vi "Nav Joystick read module.vi"(3 "error in":errorcluster) -> (7 "Forward":dbl(slide) scale=-10.0..10.0, 8 "Heading":dbl(slide) scale=-10.0..10.0, 9 "Lat":dbl(slide) scale=-10.0..10.0, 10 "error out":errorcluster)   [LabVIEW 2021]
doc: "Demonstrates how to access assembly instance data by using Explicit Messaging."
panel:
  out "Trim":u8(slide) scale=0.0..255.0
  out "Right":bool
  out "Left":bool
  out "depth":bool
  out "Dn":bool
  out "Up":bool
  out "element":u8
  out "data received":u8[](array[numeric])
  in  "network path":string="192.168.81.28"
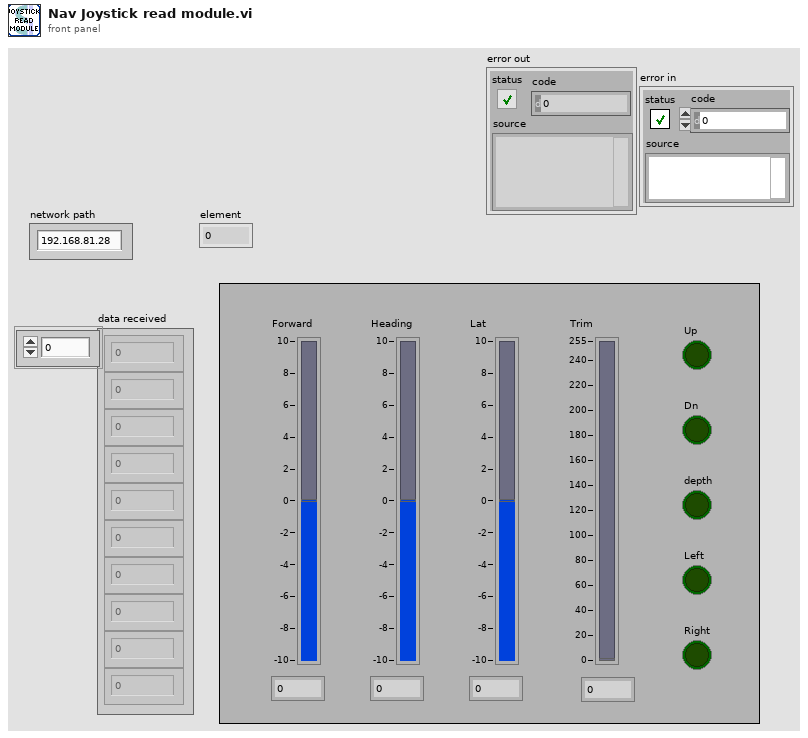
[diagram p1: front panel]
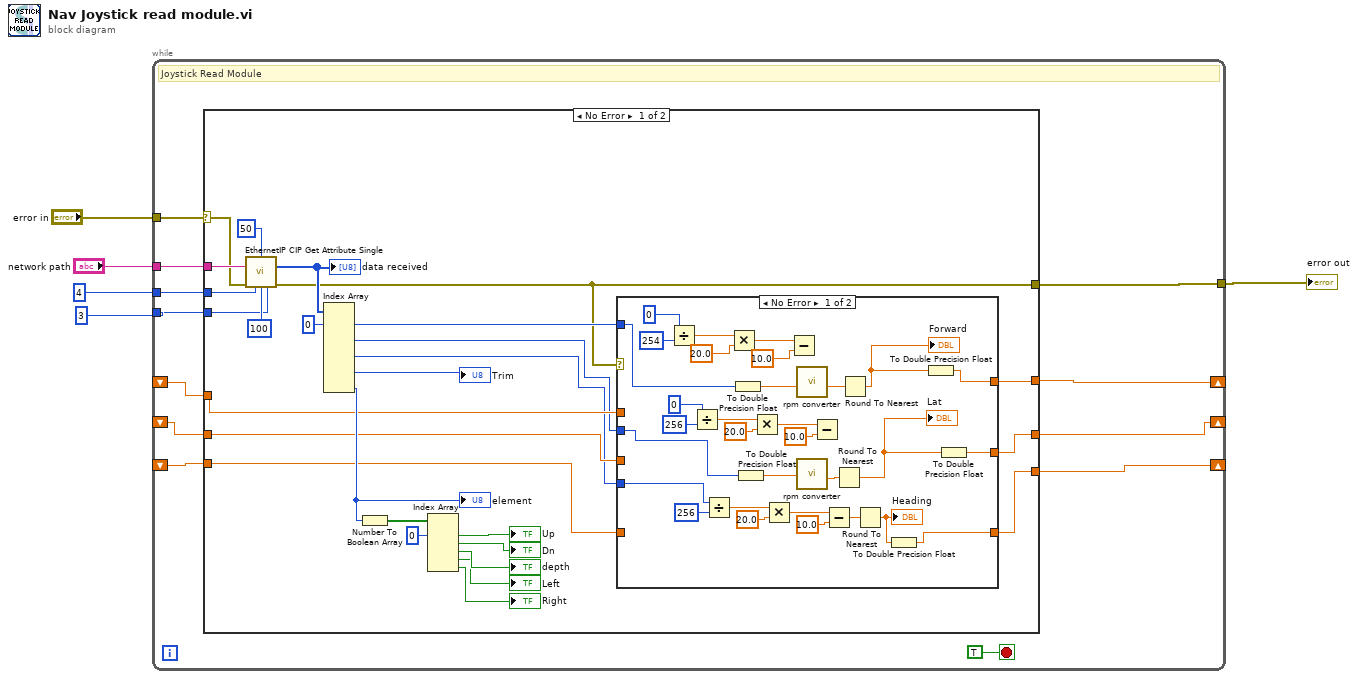
[diagram p0: block diagram]
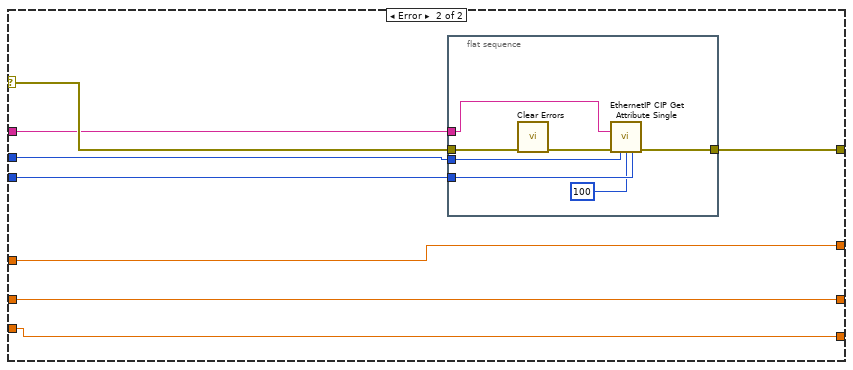
[diagram p3: hidden frame]
diagram:
  n1 = while {
    tunnel: "network path" -> [w17]
    tunnel: 4 ("Class") -> [w16]
    tunnel: 3 ("Attribute") -> [w15]
    shift-right: [w10] -> _
    shift-left: _ -> [w11]
    tunnel: "error in" -> [w12]
    tunnel: [w14] -> w2
    shift-right: [w9] -> _
    shift-left: _ -> [w8]
    shift-right: [w6] -> _
    shift-left: _ -> [w7]
    stop <- TRUE stop-if-true
    # "Joystick Read Module"
    n2 = case shown="No Error" w12 {
      selector: w12 -> [w18 w86]
      tunnel: w17 -> [w43 w84]
      tunnel: w16 -> [w42 w83]
      tunnel: w15 -> [w41 w82]
      tunnel: [w26 w85] -> w14
      tunnel: [w27 w81] -> w10
      tunnel: w11 -> [w25 w81]
      tunnel: [w24 w80] -> w9
      tunnel: w8 -> [w23 w80]
      tunnel: w7 -> [w21 w79]
      tunnel: [w20 w79] -> w6
      frame No Error {
        n3 = call <vilib>:"EthernetIP CIP Get Attribute Single.vi"("Timeout (ms)"=50 ("timeout [ms]"), "Network Path"=w43, "error in"=w18, "Class"=w42, "Instance"=u32 100 ("assembly instance ID"), "Attribute"=w41) -> ("Data"=w39:u8[], "error out"=w26:errorcluster)  [unwired: 1 in, 7 out]
        "data received" <- w39
        n4 = Index Array(array=w39, index #1=0 ("index")) -> (element #1=w28:u8, element #3=w22:u8, element #5=w19:u8, element #7=→"Trim":u8, element #9=w37:u8)  [unwired: 8 in, 4 out]
        "element" <- w37
        n5 = Number To Boolean Array(number=w37) -> (Boolean array=w36:bool[])
        n6 = Index Array(array=w36, index #1=0 ("index")) -> (element #1=→"Up":bool, element #2=→"Dn":bool, element #3=→"depth":bool, element #4=→"Left":bool, element #5=→"Right":bool)  [unwired: 4 in]
        n7 = case shown="No Error" w26 {
          tunnel: w28 -> [w51 _]
          tunnel: [w69 w78] -> w27
          tunnel: w25 -> [_ w78]
          tunnel: [w62 w77] -> w24
          tunnel: w23 -> [_ w77]
          tunnel: w22 -> [w48 _]
          tunnel: [w54 w76] -> w20
          tunnel: w21 -> [_ w76]
          tunnel: w19 -> [w53 _]
          frame No Error {
            n8 = Divide(x=0, y=254) -> (x/y=w75:dbl)
            n9 = Divide(x=0, y=256) -> (x/y=w68:dbl)
            n10 = Divide(x=w53, y=256) -> (x/y=w61:dbl)
            n11 = Multiply(x=w75, y=20.0) -> (x*y=w73:dbl)
            n12 = To Double Precision Float(number=w51) -> (double precision float=w50:dbl)
            n13 = To Double Precision Float(number=w48) -> (double precision float=w47:dbl)
            n14 = Multiply(x=w68, y=20.0) -> (x*y=w66:dbl)
            n15 = Multiply(x=w61, y=20.0) -> (x*y=w59:dbl)
            n16 = Subtract(x=w73, y=10.0) -> ()  [unwired: 1 out]
            n17 = call "rpm converter.vi"("y"=w50) -> ("x-y"=w52:dbl)  [unwired: 10 in]
            n18 = call "rpm converter.vi"("y"=w47) -> ("x-y"=w45:dbl)  [unwired: 10 in]
            n19 = Subtract(x=w66, y=10.0) -> ()  [unwired: 1 out]
            n20 = Subtract(x=w59, y=10.0) -> (x-y=w57:dbl)
            n21 = Round To Nearest(number=w45) -> (nearest integer value=w64:dbl)
            "Lat" <- w64
            n22 = Round To Nearest(number=w52) -> (nearest integer value=w71:dbl)
            "Forward" <- w71
            n23 = Round To Nearest(number=w57) -> (nearest integer value=w56:dbl)
            "Heading" <- w56
            n24 = To Double Precision Float(number=w56) -> (double precision float=w54:dbl)
            n25 = To Double Precision Float(number=w71) -> (double precision float=w69:dbl)
            n26 = To Double Precision Float(number=w64) -> (double precision float=w62:dbl)
          }
          frame Error {
          }
        }
      }
      frame Error {
        n27 = flat-sequence {
          tunnel: w86 -> [w93]
          tunnel: [w91] -> w85
          tunnel: w84 -> [w90]
          tunnel: w83 -> [w89]
          tunnel: w82 -> [w88]
          frame #0 {
            n28 = call <vilib>:"Clear Errors.vi"("error in (no error)"=w93) -> ("error out"=w92:errorcluster)  [unwired: 5 in, 1 out]
            n29 = call <vilib>:"EthernetIP CIP Get Attribute Single.vi"("Network Path"=w90, "error in"=w92, "Class"=w89, "Instance"=u32 100, "Attribute"=w88) -> ("error out"=w91:errorcluster)  [unwired: 2 in, 8 out]
          }
        }
      }
    }
  }
  "error out" <- w2
